vi "HitrapGUI.HTLE_TR7.vi"() -> ()   [LabVIEW 2014, in "HitrapGUI.lvlib"]
uses:
  HitrapGUI.lvlib
  CSlibraries/GUILib/GUILib.userEventsMainType.ctl
  CSlibraries-extern/DimLVEvent/DimIndicators/DimIndicators.anyType.ctl
  CSlibraries/GUILib/GUILib.simpleNumeric.ctl
  CSlibraries/GUILib/GUILib.basicNumeric.ctl
  CSlibraries/UtilityLib/UtilityLib.valueStatus.ctl
  CS_Core/CSSystem/CoreDefs/CoreDefs.rawDataType.ctl
  CS_Core/CSSystem/CoreLib/CoreLib.double 2 byte array.vi
  CSlibraries/UtilityLib/UtilityLib.lvlib
  CS_Core/CSSystem/CSSystemLib/CSSystemLib.lvlib
  CSlibraries-extern/DimLVEvent/DimIndicators/DimIndicators.lvlib
  CS_Core/GUIs/GOGControllerGUI/GOGControllerGUI.lvlib
  CSlibraries/GUILib/GUILib.lvlib
  CS_Core/CSSystem/CoreLib/CoreLib.lvlib
panel:
  in  "TR7QD1_4":bool=TRUE
  in  "TR7QD1_3":bool=TRUE
  in  "TR7QD1_2":bool=TRUE
  in  "TR7QD1_4Ctl":T1 {"nom" step=1.0}
  in  "TR7QD1_3Ctl":T1 {"nom" step=1.0}
  in  "TR7QD1_2Ctl":T1 {"nom" step=1.0}
  in  "TR7QD1_1Ctl":T1 {"nom" step=1.0}
  in  "TR7QD1_1":bool=TRUE
  in  "TR6QD5_4Ctl":T1 {"nom" step=1.0}
  in  "TR6QD5_4":bool=TRUE
  in  "TR6QD5_3Ctl":T1 {"nom" step=1.0}
  in  "TR6QD5_3":bool=TRUE
  in  "TR6QD5_2Ctl":T1 {"nom" step=1.0}
  in  "TR6QD5_2":bool=TRUE
  in  "TR6QD5_1Ctl":T1 {"nom" step=1.0}
  in  "TR6QD5_1":bool=TRUE
  out "subSystem6State":string
  in  "subSystem1":bool
  out "subSystem6StateQuality":string
  in  "subControllersIgnoredDIM":T3
  in  "iniData":string
  in  "stop":bool
  in  "dummy":bool
  in  "parentSystem":bool
  in  "userEvent":refnum<user-event>
  # "TR7"
  # "(Platform, EBIT)"
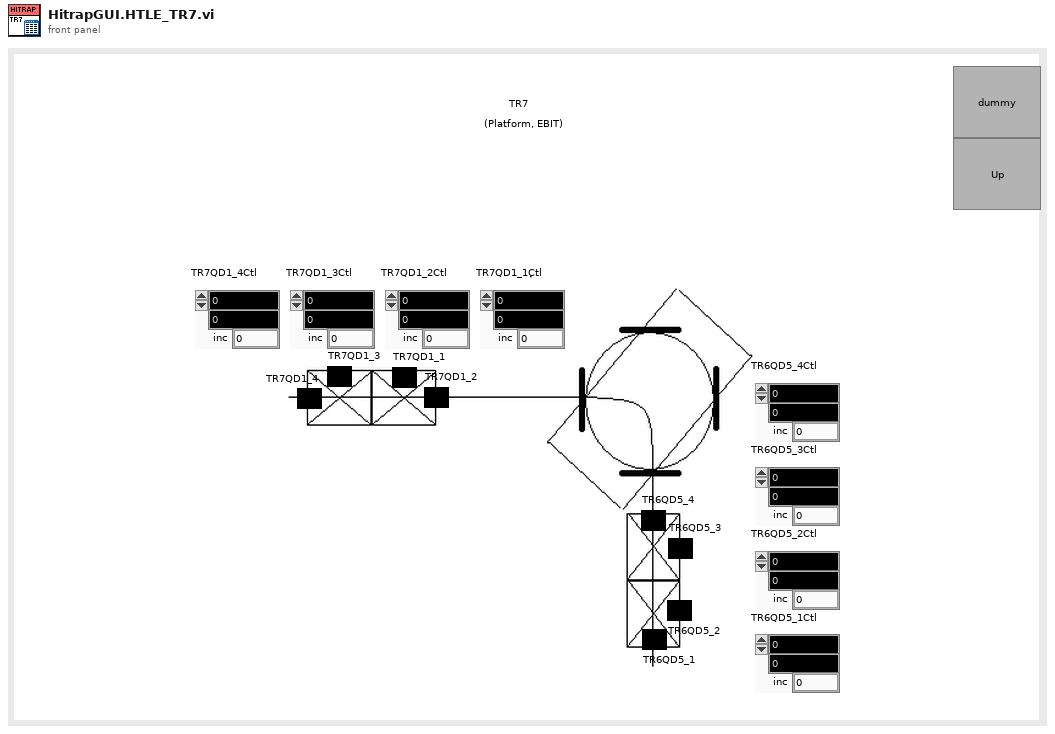
[diagram p1: front panel]
types:
  T1 = typedef "GUILib.lvlib/GUILib.simpleNumeric.ctl" = cluster{"nom":T2, "act":dbl, "inc":dbl}
  T2 = typedef "GUILib.lvlib/GUILib.basicNumeric.ctl" = dbl
  T3 = typedef "DimIndicators.lvlib/DimIndicators.anyType.ctl" = cluster{"data":string, "no link":bool, "quality":i32, "timeStamp":dbl}
  T4 = typedef "UtilityLib.lvlib/UtilityLib.valueStatus.ctl" = enum16{"no info available", "stand by/off", "on", "warning", "alarm/malfunction", "not implemented", "user action required", "important information", "system default", "control default", "indicator default", "button default"}
  T5 = typedef "CoreDefs.rawDataType.ctl" = i8[]
  T6 = typedef "lveventtype.ctl" = enum32{"Null", "Timeout", "Annotation Menu Selection", "Annotation Menu Selection?", "App Instance Close", "App Instance Close?", "Autoscale Range Change", "Bookmark Info Change", "Cell Edit", "Cell Edit?", "Cursor Grab", "Cursor Grab?", "Cursor Menu Selection", "Cursor Menu Selection?", "Cursor Move", "Cursor Release", "Data Change", "Direction Change", "Display State Change", "Drag Ended", "Drag Enter", "Drag Leave", "Drag Over", "Drag Source Update", "Drag Starting", "Drag Starting?", "Drop", "Exec State Change", "Key Down", "Key Down?", "Key Repeat", "Key Repeat?", "Key Up", "Listbox Double Click", "Menu Activation?", "Menu Selection (App)", "Menu Selection? (App)", "Menu Selection (User)", "Mouse Down", "Mouse Down?", "Mouse Enter", "Mouse Leave", "Mouse Move", "Mouse Up", "Mouse Wheel", "NI Security User Change (App)", "Pane Size", "Panel Close", "Panel Close?", "Panel Resize", "Plot Attribute Change", "Scale Range Change", "Shortcut Menu Activation?", "Shortcut Menu Selection (App)", "Shortcut Menu Selection? (App)", "Shortcut Menu Selection (User)", "Tree Double Click", "Tree Drag", "Tree Drag?", "Tree Drop", "Tree Drop?", "Tree Item Close", "Tree Item Close?", "Tree Item Open", "Tree Item Open?", "User Event", "Value Change"}
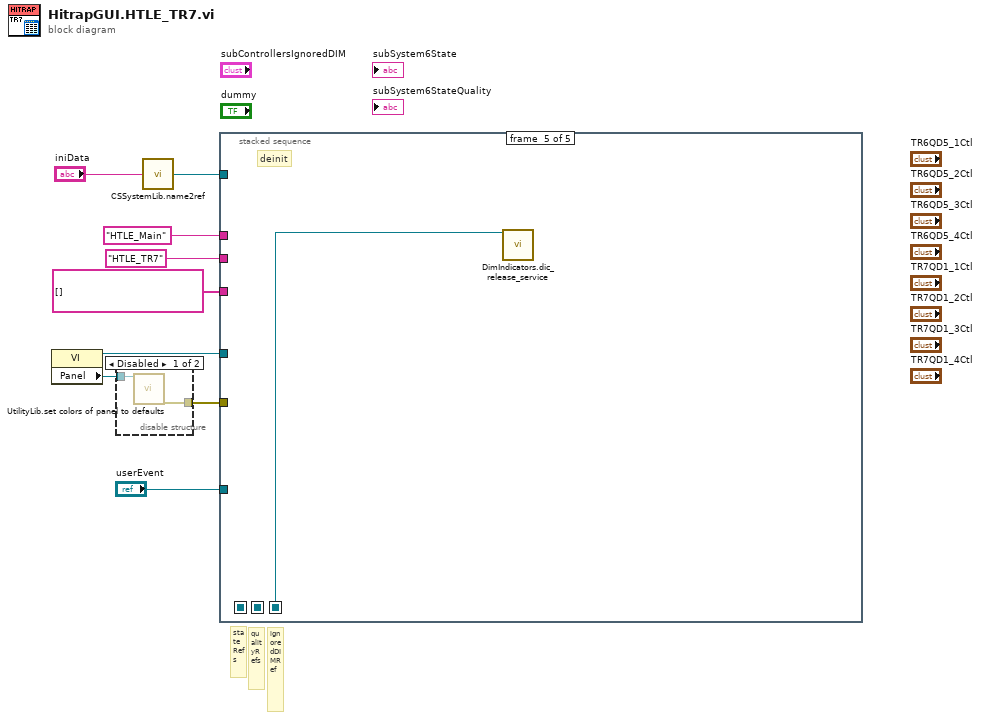
[diagram p0: block diagram]
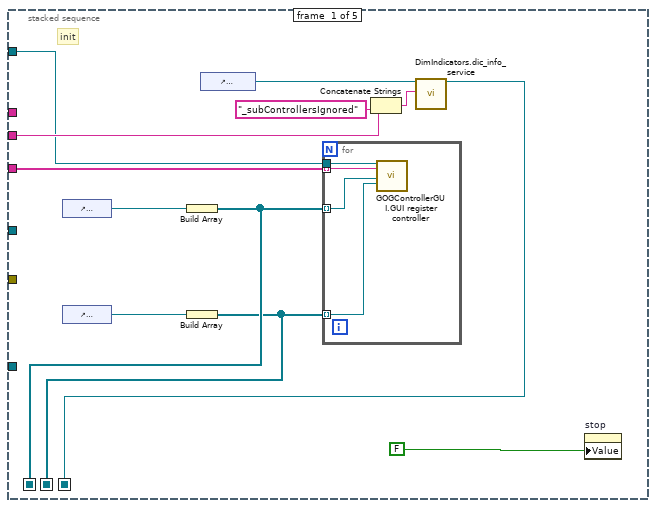
[diagram p3: hidden frame]
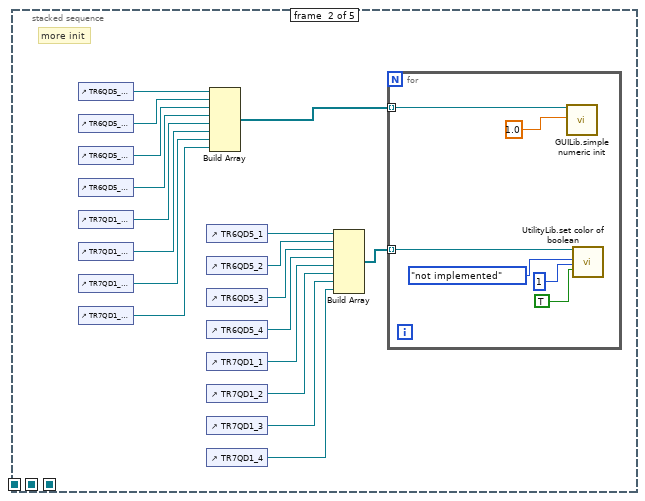
[diagram p4: hidden frame]
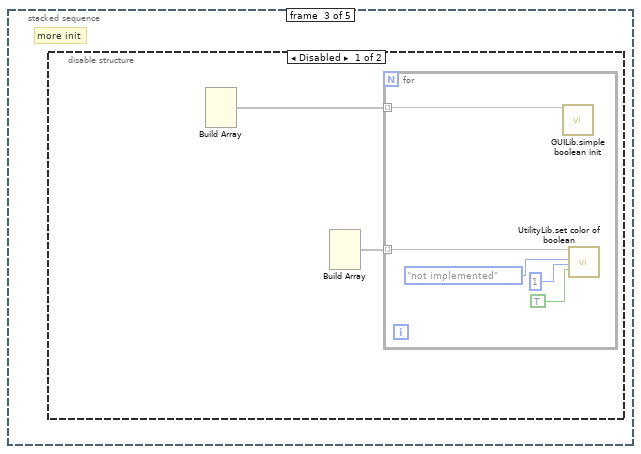
[diagram p5: hidden frame]
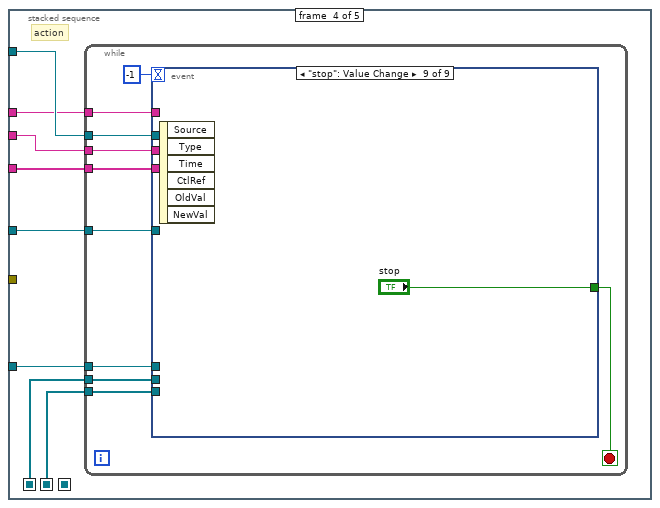
[diagram p7: hidden frame]
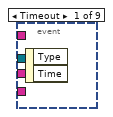
[diagram p8: hidden frame]
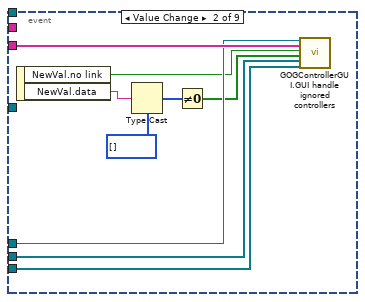
[diagram p9: hidden frame]
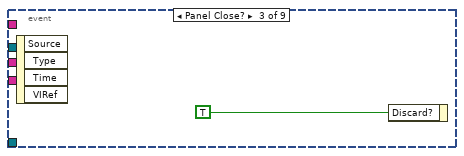
[diagram p10: hidden frame]
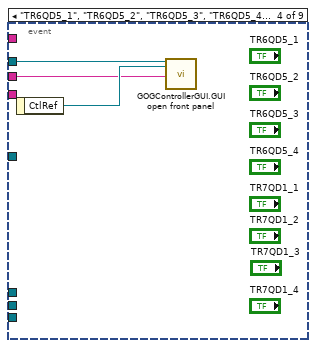
[diagram p11: hidden frame]
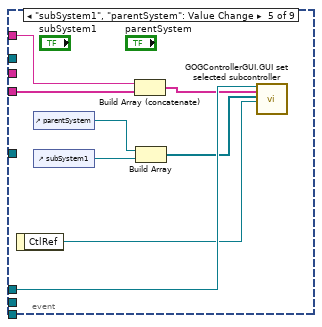
[diagram p12: hidden frame]
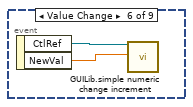
[diagram p13: hidden frame]
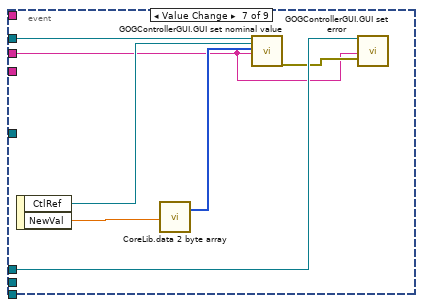
[diagram p14: hidden frame]
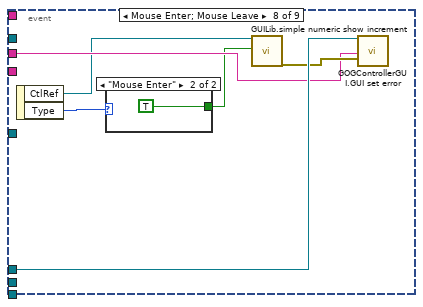
[diagram p15: hidden frame]
diagram:
  # "qualityRefs"
  # "ignoredDIMRef"
  # "stateRefs"
  n1 = property class="VI"() -> (reference out=w7:refnum<vi>, "Panel"=w8:refnum<vi>)  [unwired: 2 in, 1 out]
  n2 = disable-structure shown="Disabled" {
    disable-tunnel: w8 -> [w11 _]
    disable-tunnel: [w10 _] -> w6
    frame Disabled {
      n3 = call "UtilityLib.set colors of panel to defaults.vi"("Front Panel"=w11) -> ("error out"=w10:errorcluster)  [unwired: 18 in]
    }
    frame Enabled {
    }
  }
  n4 = call "CSSystemLib.name2ref.vi"("name"="iniData") -> ("obj refnum"=w2:refnum<vi>)
  n5 = stacked-sequence {
    seq-local: [w13 _ _ _ _] -> [_ _ _ _ w125]
    seq-local: [w14 _ _ _ _] -> [_ _ _ w73 _]
    seq-local: [w12 _ _ _ _] -> [_ _ _ w72 _]
    tunnel: "userEvent" -> [_ _ _ w76 _]
    tunnel: w7 -> [_ _ _ w75 _]
    tunnel: w6 -> [_ _ _ _ _]
    tunnel: "HTLE_TR7" -> [w19 _ _ w70 _]
    tunnel: string[] [] -> [w18 _ _ w74 _]
    tunnel: w2 -> [w17 _ _ w71 _]
    tunnel: "HTLE_Main" -> [_ _ _ w69 _]
    frame #0 {
      # "init"
      n6 = control-ref of="dummySubSystemState"() -> (w16:refnum<vi>)
      n7 = control-ref of="dummySubSystemStateQuality"() -> (w15:refnum<vi>)
      n8 = Build Array(w16) -> (w14:refnum<vi>[])
      n9 = Build Array(w15) -> (w12:refnum<vi>[])
      n10 = control-ref of="subControllersIgnoredDIM"() -> (w20:refnum<vi>)
      n11 = for {
        tunnel: w14 -> [w27] mode=indexing
        tunnel: w18 -> [w25] mode=indexing
        tunnel: w12 -> [w24] mode=indexing
        tunnel: w17 -> [w26]
        n12 = call "GOGControllerGUI.GUI register controller.vi"("i ref in"=w26, "controllerName"=w25, "subSystemState"=w27, "subSystemStateQuality"=w24) -> ()  [unwired: 14 in, 2 out]
      }
      n13 = Concatenate Strings(w19, "_subControllersIgnored" ("string")) -> (w22:string)
      n14 = call "DimIndicators.dic_info_service.vi"("controlRef"=w20, "serviceName"=w22) -> ("controlRef out"=w13:refnum<vi>)  [unwired: 16 in, 1 out]
      n15 = property on="stop" class="Bool (strict)"("Value"=FALSE ("stop")) -> ()  [unwired: 2 in, 2 out]
    }
    frame #1 {
      # "more init"
      n16 = control-ref of="TR6QD5_1Ctl"() -> (w45:refnum<vi>)
      n17 = control-ref of="TR6QD5_2Ctl"() -> (w44:refnum<vi>)
      n18 = control-ref of="TR6QD5_3Ctl"() -> (w43:refnum<vi>)
      n19 = control-ref of="TR6QD5_4Ctl"() -> (w42:refnum<vi>)
      n20 = control-ref of="TR7QD1_1Ctl"() -> (w41:refnum<vi>)
      n21 = control-ref of="TR7QD1_2Ctl"() -> (w33:refnum<vi>)
      n22 = control-ref of="TR7QD1_3Ctl"() -> (w32:refnum<vi>)
      n23 = control-ref of="TR7QD1_4Ctl"() -> (w31:refnum<vi>)
      n24 = control-ref of="TR6QD5_1"() -> (w39:refnum<vi>)
      n25 = control-ref of="TR6QD5_2"() -> (w38:refnum<vi>)
      n26 = control-ref of="TR6QD5_3"() -> (w37:refnum<vi>)
      n27 = control-ref of="TR6QD5_4"() -> (w36:refnum<vi>)
      n28 = control-ref of="TR7QD1_1"() -> (w35:refnum<vi>)
      n29 = control-ref of="TR7QD1_2"() -> (w30:refnum<vi>)
      n30 = control-ref of="TR7QD1_3"() -> (w29:refnum<vi>)
      n31 = control-ref of="TR7QD1_4"() -> (w28:refnum<vi>)
      n32 = Build Array(w45, w44, w43, w42, w41, w33, w32, w31) -> (w40:refnum<vi>[])
      n33 = Build Array(w39, w38, w37, w36, w35, w30, w29, w28) -> (w34:refnum<vi>[])
      n34 = for {
        tunnel: w40 -> [w51] mode=indexing
        tunnel: w34 -> [w47] mode=indexing
        n35 = call "GUILib.simple numeric init.vi"("ctlRef"=w51, "increment"=1.0) -> ()  [unwired: 16 in, 2 out]
        n36 = call "UtilityLib.set color of boolean.vi"("button"=w47, "valueStatus"=UtilityLib.valueStatus."not implemented", "nOfPair (0)"=1, "setTRUEColor (FALSE)"=TRUE) -> ()  [unwired: 15 in, 1 out]
      }
    }
    frame #2 {
      # "more init"
      n37 = disable-structure shown="Disabled" {
        frame Disabled {
          n38 = Build Array() -> (w58:void[], w63:dbl, w62:dbl, w61:dbl, w60:dbl, w59:dbl)
          n39 = Build Array() -> (w52:void[], w57:dbl, w56:dbl, w55:dbl, w54:dbl, w53:dbl)
          n40 = for {
            tunnel: w58 -> [w68] mode=indexing
            tunnel: w52 -> [w64] mode=indexing
            n41 = call "GUILib.simple boolean init.vi"("ctlRef"=w68) -> ()  [unwired: 17 in, 2 out]
            n42 = call "UtilityLib.set color of boolean.vi"("button"=w64, "valueStatus"=UtilityLib.valueStatus."not implemented", "nOfPair (0)"=1, "setTRUEColor (FALSE)"=TRUE) -> ()  [unwired: 15 in, 1 out]
          }
        }
        frame Enabled {
        }
      }
    }
    frame #3 {
      # "action"
      n43 = while {
        tunnel: w76 -> [w86]
        tunnel: w75 -> [w84]
        tunnel: w74 -> [w82]
        tunnel: w73 -> [w81]
        tunnel: w72 -> [w80]
        tunnel: w71 -> [w79]
        tunnel: w70 -> [w78]
        tunnel: w69 -> [w77]
        stop <- w83 stop-if-true
        n44 = event shown="[8] \"stop\": Value Change" {
          selector: _ -> [_ _ _ _ _ _ _ _ _]
          dyn-events: _ -> [_ _ _ _ _ _ _ _ _]
          timeout: -1 -> [_ _ _ _ _ _ _ _ _]
          tunnel: w86 -> [_ w91 _ _ w106 _ w112 w122 _]
          tunnel: w84 -> [_ _ _ _ _ _ _ _ _]
          tunnel: [_ _ _ _ _ _ _ _ "stop"] -> w83
          tunnel: w82 -> [_ w92 _ _ w102 _ _ _ _]
          tunnel: w81 -> [_ w88 _ _ _ _ _ _ _]
          tunnel: w80 -> [_ w87 _ _ _ _ _ _ _]
          tunnel: w79 -> [_ _ _ w99 _ _ w116 _ _]
          tunnel: w78 -> [_ _ _ w97 _ _ w110 w120 _]
          tunnel: w77 -> [_ _ _ _ w101 _ _ _ _]
          event Timeout {
            n45 = event-data() -> ()  [unwired: 1 in, 2 out]
          }
          event Value Change {
            n46 = event-data() -> ("NewVal.no link"=w90:bool, "NewVal.data"=w93:string)  [unwired: 1 in]
            n47 = Type Cast(type=T5 [] ("Array"), x=w93) -> (*(type *) &x=w95:T5)
            n48 = Not Equal To 0?(x=w95) -> (x != 0?=w89:bool[])
            n49 = call "GOGControllerGUI.GUI handle ignored controllers.vi"("userEvent"=w91, "controllerNames"=w92, "NOLINK"=w90, "controllersIgnored"=w89, "stateRefs"=w88, "qualityRefs"=w87) -> ()  [unwired: 14 in]
          }
          event Panel Close? {
            n50 = event-data() -> ()  [unwired: 1 in, 4 out]
            n51 = event-data("Discard?"=TRUE) -> ()  [unwired: 1 in, 1 out]
          }
          event "TR6QD5_1", "TR6QD5_2", "TR6QD5_3", "TR6QD5_4", "TR7QD1_1", "TR7QD1_2", "TR7QD1_3", "TR7QD1_4": Value Change {
            n52 = event-data() -> ("CtlRef"=w98:refnum<vi>)  [unwired: 1 in]
            n53 = call "GOGControllerGUI.GUI open front panel.vi"("i ref in"=w99, "elementRef"=w98, "controller"=w97) -> ()  [unwired: 15 in, 2 out]
          }
          event "subSystem1", "parentSystem": Value Change {
            n54 = event-data() -> ("CtlRef"=w104:refnum<vi>)  [unwired: 1 in]
            n55 = control-ref of="parentSystem"() -> (w103:refnum<vi>)
            n56 = control-ref of="subSystem1"() -> (w107:refnum<vi>)
            n57 = Build Array (concatenate)(w101, w102) -> (w100:string[])
            n58 = Build Array(w103, w107) -> (w105:refnum<vi>[])
            n59 = call "GOGControllerGUI.GUI set selected subcontroller.vi"("userEvent"=w106, "controllerNames"=w100, "controllerRefs"=w105, "controllerRef"=w104) -> ()  [unwired: 16 in]
          }
          event Value Change {
            n60 = event-data() -> ("CtlRef"=w109:refnum<vi>, "NewVal"=w108:dbl)  [unwired: 1 in]
            n61 = call "GUILib.simple numeric change increment.vi"("ctlRef"=w109, "increment"=w108) -> ()  [unwired: 16 in, 2 out]
          }
          event Value Change {
            n62 = event-data() -> ("CtlRef"=w115:refnum<vi>, "NewVal"=w114:T2)  [unwired: 1 in]
            n63 = call-poly "CoreLib.data 2 byte array.vi"("f64"=w114) -> ("byteArray out"=w113:T5)  [unwired: 18 in]
            n64 = call "GOGControllerGUI.GUI set nominal value.vi"("i ref in"=w116, "nominalRef"=w115, "nominalData"=w113, "controller"=w110) -> ("error out"=w111:errorcluster)  [unwired: 14 in, 1 out]
            n65 = call "GOGControllerGUI.GUI set error.vi"("userEvent"=w112, "controller"=w110, "GUIError"=w111) -> ()  [unwired: 16 in, 1 out]
          }
          event Mouse Enter; Mouse Leave {
            n66 = event-data() -> ("CtlRef"=w119:refnum<vi>, "Type"=w118:T6)  [unwired: 1 in]
            n67 = case shown="\"Mouse Enter\"" w118 {
              tunnel: [_ TRUE] -> w117
              frame Default {
              }
              frame "Mouse Enter" {
              }
            }
            n68 = call "GUILib.simple numeric show increment.vi"("ctlRef"=w119, "show"=w117) -> ("error out"=w121:errorcluster)  [unwired: 16 in, 1 out]
            n69 = call "GOGControllerGUI.GUI set error.vi"("userEvent"=w122, "controller"=w120, "GUIError"=w121) -> ()  [unwired: 16 in, 1 out]
          }
          event "stop": Value Change {
            n70 = event-data() -> ()  [unwired: 1 in, 6 out]
          }
        }
      }
    }
    frame #4 {
      # "deinit"
      n71 = call "DimIndicators.dic_release_service.vi"("controlRef"=w125) -> ()  [unwired: 18 in, 1 out]
    }
  }
